vi "Open Front Panel.vi"(8 "error in (no error)":errorcluster, 11 "Cursor Digitizer in":refnum<class "Cursor Digitizer.lvclass">) -> (0 "error out":errorcluster, 3 "Cursor Digitizer out":refnum<class "Cursor Digitizer.lvclass">)   [LabVIEW 2016, in "Cursor Digitizer.lvclass"]
uses:
  Cursor Digitizer.lvclass
  Cursor Digitizer.lvclass/Cursor Digitizer.ctl
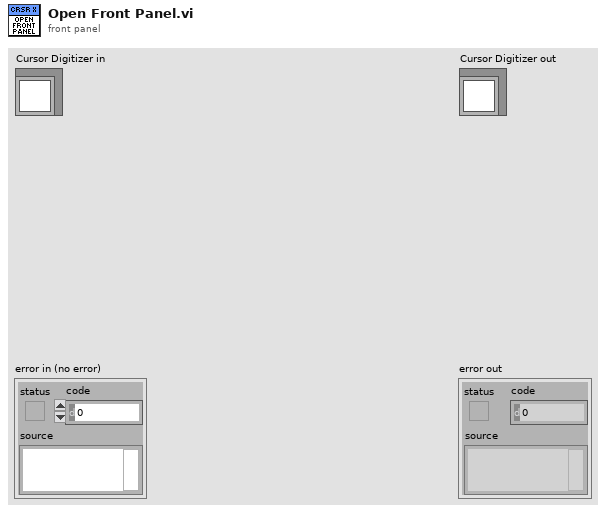
[diagram p1: front panel]
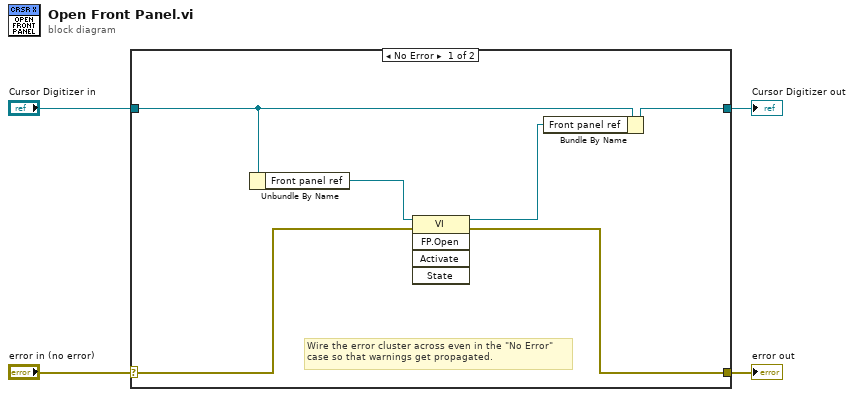
[diagram p0: block diagram]
diagram:
  n1 = case shown="No Error" "error in (no error)" {
    selector: "error in (no error)" -> [w8 w12]
    tunnel: [w7 w12] -> w3
    tunnel: [w6 w11] -> w1
    tunnel: "Cursor Digitizer in" -> [w10 w11]
    frame No Error {
      # "Wire the error cluster across even in the \"No Error\"\ncase so that warnings get propagated."
      n2 = Unbundle By Name(w10) -> ("Front panel ref"=w9:refnum<vi>)
      n3 = invoke class="VI" method="FP.Open"(reference=w9, error in=w8) -> (reference out=w5:refnum<vi>, error out=w7:errorcluster)  [unwired: 3 in, 3 out]
      n4 = Bundle By Name(cluster=w10, "Front panel ref"=w5) -> (w6:refnum<class "Cursor Digitizer.lvclass">)
    }
    frame Error {
    }
  }
  "error out" <- w3
  "Cursor Digitizer out" <- w1
